vi "Get Result Events.vi"(8 "error in (no error)":errorcluster, 11 "event_input in":refnum<class "event_input.lvclass">) -> (0 "error out":errorcluster, 2 "result_event":refnum<user-event>, 3 "event_input out":refnum<class "event_input.lvclass">)   [LabVIEW 2015, in "event_input.lvclass"]
uses:
  event_input.lvclass
  result/result.lvclass
  event_input.lvclass/event_input.ctl
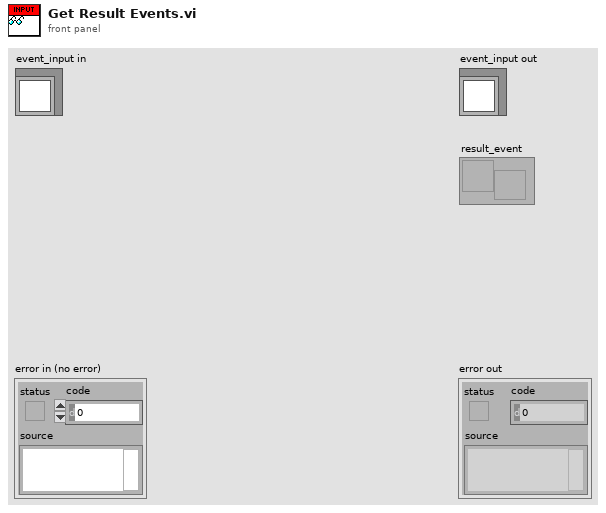
[diagram p1: front panel]
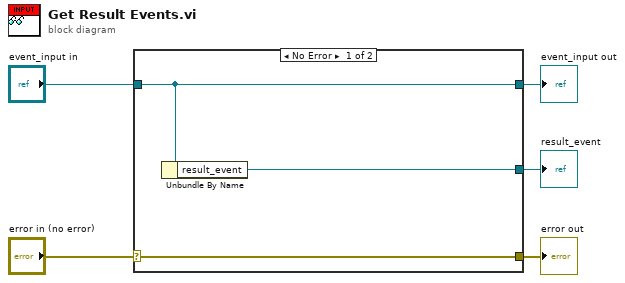
[diagram p0: block diagram]
diagram:
  n1 = case shown="No Error" "error in (no error)" {
    selector: "error in (no error)" -> [w8 w9]
    tunnel: [w8 w9] -> w4
    tunnel: [w7 w10] -> w2
    tunnel: "event_input in" -> [w7 w10]
    tunnel: [w6 _] -> w1
    frame No Error {
      n2 = Unbundle By Name(w7) -> ("result_event"=w6:refnum<user-event>)
    }
    frame Error {
    }
  }
  "error out" <- w4
  "event_input out" <- w2
  "result_event" <- w1
